vi "Write_Data.vi"(10 "Secondary Parameter":dbl, 11 "Primary Parameter":dbl) -> (3 "String":string)   [LabVIEW 2017]
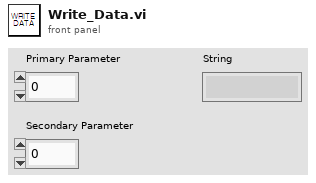
[diagram p1: front panel]
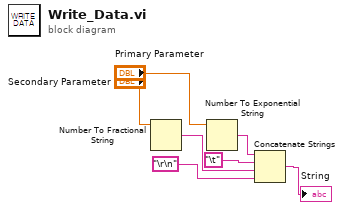
[diagram p0: block diagram]
diagram:
  n1 = Number To Fractional String(number="Secondary Parameter") -> (F-format string=w2:string)  [unwired: 3 in]
  n2 = Number To Exponential String(number="Primary Parameter") -> (E-format string=w6:string)  [unwired: 3 in]
  n3 = Concatenate Strings(w6, "\t", w2, "\r\n") -> (→"String":string)
